vi "Read Power.vi"(8 "error in":errorcluster, 11 "Change Meerstetter Power in":refnum<class "Change Meerstetter Power.lvclass">) -> (0 "error out":errorcluster, 2 "Power":sgl, 3 "Change Meerstetter Power out":refnum<class "Change Meerstetter Power.lvclass">)   [LabVIEW 2014, in "Meerstetter Lib.lvlib" / "Change Meerstetter Power.lvclass"]
uses:
  Change Meerstetter Power.lvclass
  Change Meerstetter Power.lvclass/Change Meerstetter Power.ctl
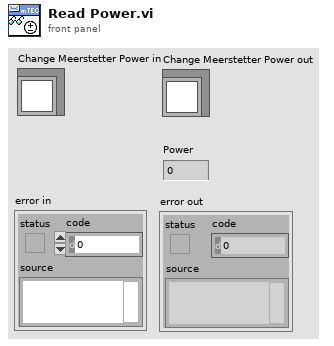
[diagram p1: front panel]
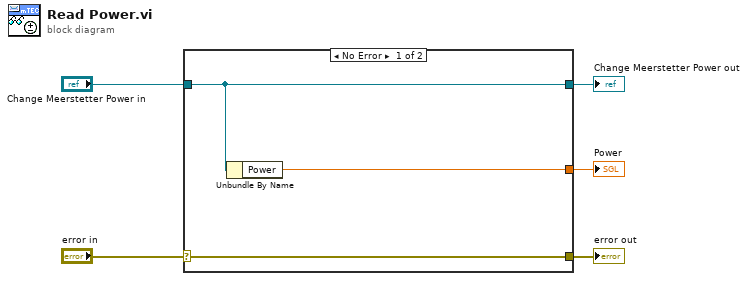
[diagram p0: block diagram]
diagram:
  n1 = case shown="No Error" "error in" {
    selector: "error in" -> [w8 w9]
    tunnel: [w8 w9] -> w4
    tunnel: [w7 w10] -> w2
    tunnel: "Change Meerstetter Power in" -> [w7 w10]
    tunnel: [w6 _] -> w1
    frame No Error {
      n2 = Unbundle By Name(w7) -> ("Power"=w6:sgl)
    }
    frame Error {
    }
  }
  "error out" <- w4
  "Change Meerstetter Power out" <- w2
  "Power" <- w1
